vi "Read Worker.vi"(8 "error in (no error)":errorcluster, 11 "Worker Test in":refnum<class "Worker Test.lvclass">) -> (0 "error out":errorcluster, 2 "Worker":refnum<class "Worker.lvclass">, 3 "Worker Test out":refnum<class "Worker Test.lvclass">)   [LabVIEW 2020, in "Worker Test.lvclass"]
uses:
  Worker Test.lvclass
  Worker Test.lvclass/Worker Test.ctl
  Processes/People/Workers/Worker/Worker.lvclass
  Person Test/Person Test.lvclass
  C:/git/astemes-triarc-examples/source/Coffee Shop/Tests/Person Test/Person Test.lvclass
  C:/Program Files (x86)/National Instruments/LabVIEW 2020/vi.lib/astemes/LUnit Test Inheritance/LUnit Inheriting Test Case.lvclass
  C:/Program Files (x86)/National Instruments/LabVIEW 2020/vi.lib/Astemes/LUnit/Test Case.lvclass
  C:/Program Files (x86)/National Instruments/LabVIEW 2020/vi.lib/Astemes/LUnit/LUnit Runnable.lvclass
  C:/git/astemes-triarc-examples/source/Coffee Shop/Tests/Worker Test/Worker Test.lvclass
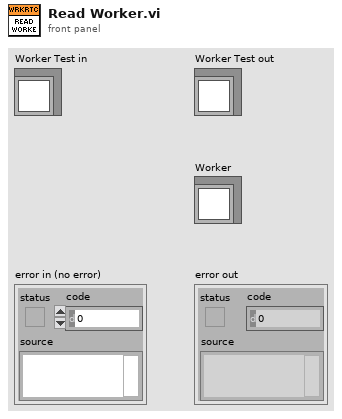
[diagram p1: front panel]
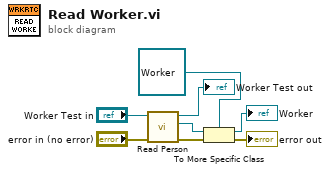
[diagram p0: block diagram]
diagram:
  n1 = call "Read Person.vi"("error in (no error)"="error in (no error)", "Person Test in"="Worker Test in") -> ("error out"=w8:errorcluster, "Person.lvclass"=w7:refnum<class "Person.lvclass">, "Person Test out"=→"Worker Test out":refnum<class "Worker Test.lvclass">)  [unwired: 7 in]
  n2 = To More Specific Class(target class=refnum<class "Worker.lvclass"> refnum ("Worker.lvclass"), reference=w7, error in=w8) -> (specific class reference=→"Worker":refnum<class "Worker.lvclass">, error out=→"error out":errorcluster)
